vi "EAGLE GUI V3.vi"() -> ()   [LabVIEW 2015]
panel:
  in  "Tab Control":enum32{"Page 1", "Page 2", "Page 3"}(tab)
  in  "NewProcedure":bool caption="Boolean"
  in  "Ready":bool caption="Boolean"
  in  "EditRout":bool caption="Boolean"
  in  "Ready 2":bool caption="Boolean"
  in  "TabSelect":T1(radio)
  in  "Tab":enum32{"Page 1", "Page 2", "Page 3"}(tab)
  in  "EyeColor":u16(ring) caption="Eye Color:" items=["Brown", "Green", "Blue", "Black"]
  in  "SysLogPath":path caption="System Log Path:"
  in  "VideoPath":path caption="Video Output Path:"
  in  "PatientGender":enum32{"Male", "Female"}(radio) caption="Patient Gender:"
  in  "PatientAge":dbl caption="Patient Age:"
  in  "PatientName":string caption="Patient Name:"
  in  "Freeze":bool caption="Boolean"
  in  "Record":bool caption="Boolean"
  out "ProcStat":string caption="Procedure Data"
  out "SystemStatus":string caption="System Status"
  in  "OpenMenu":bool
  in  "Live Eye Image":T2(plugin-control)
  in  "Procedure Instructions":T3(ring)
  # "Aim the pupil to the center of the image\nMake sure the focus laser is in the \nbar Center"
  # "When Ready Press the GO Button"
  # "Procedure Parameters"
  # "System Configuration"
  # "Patient Statistics"
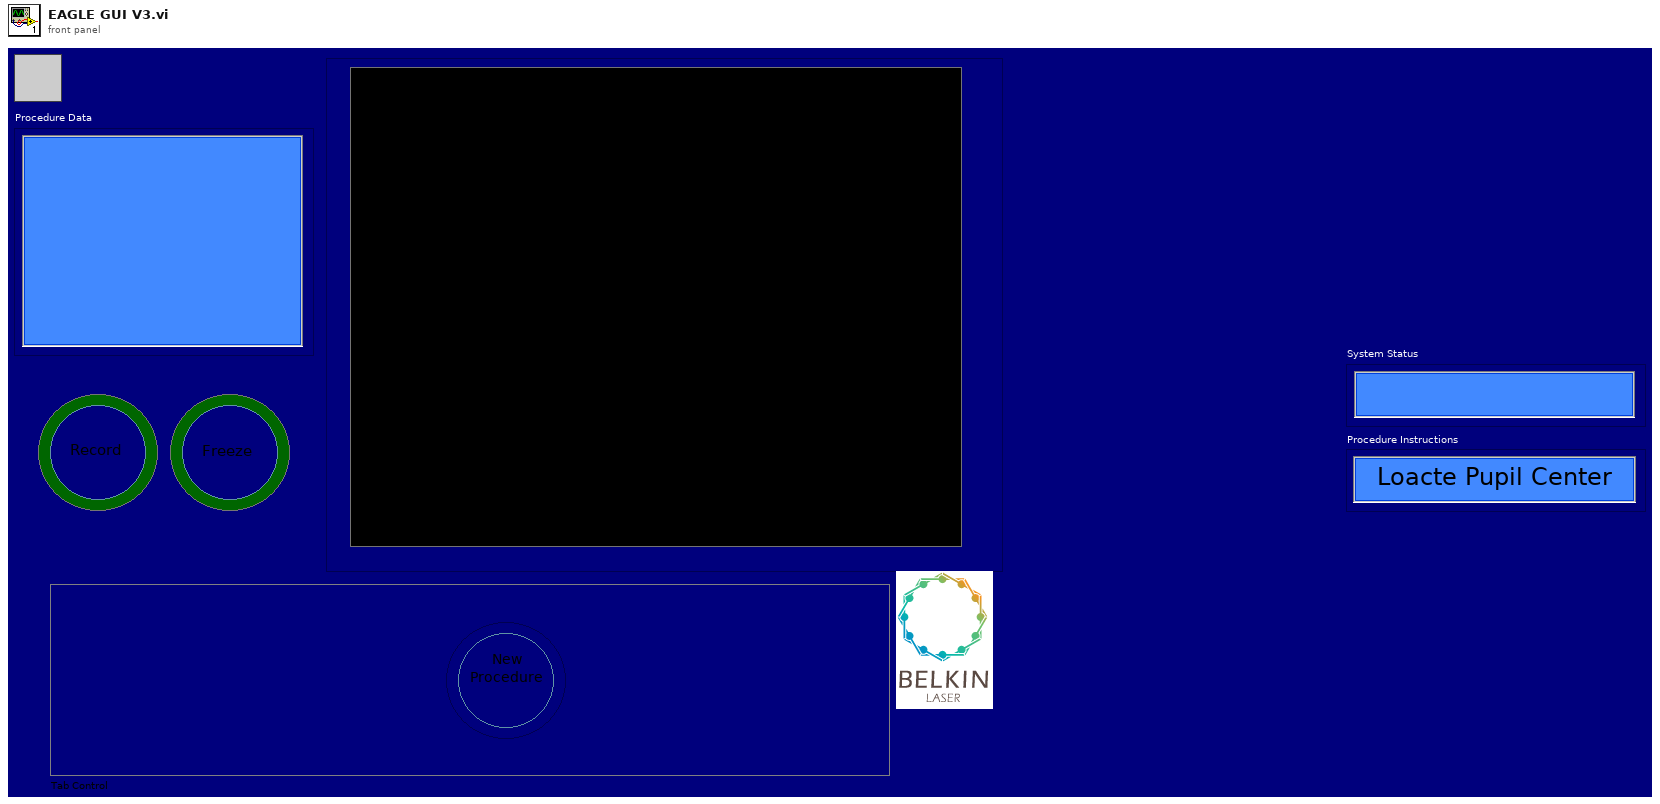
[diagram p1: front panel]
types:
  T1 = enum32{"Radio Selection 1", "Radio Selection 2", "Radio Selection 3"}
  T2 = typedef "IMAQ Image.ctl" = refnum<image>
  T3 = enum16{"Loacte Pupil Center", "Refine Distance", "CLick GO", "Process Finished"}
  T4 = typedef "LVRectTypeDef.ctl" = cluster{"Left":i16, "Top":i16, "Right":i16, "Bottom":i16}
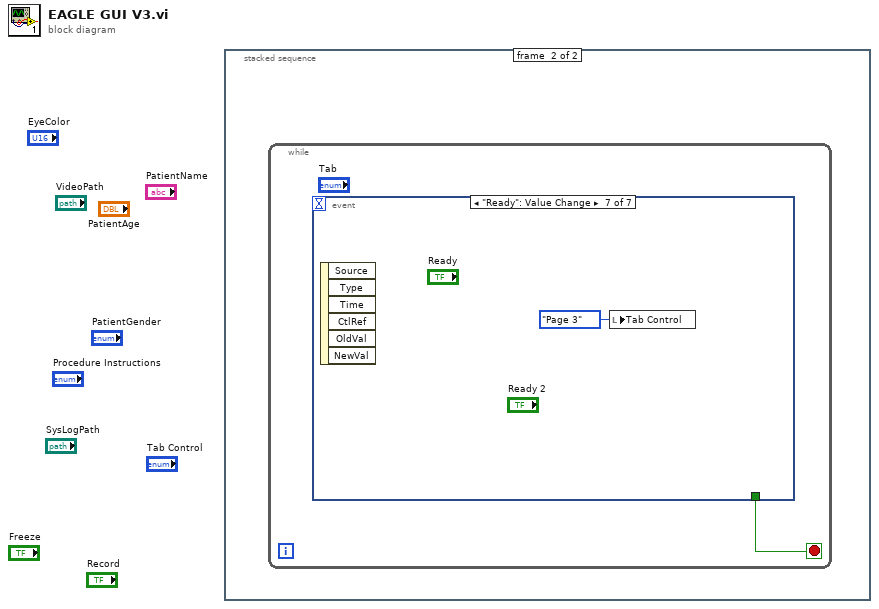
[diagram p0: block diagram]
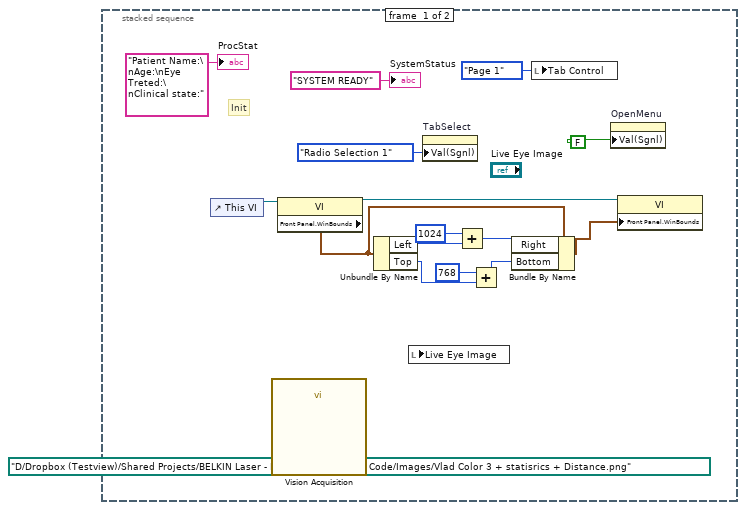
[diagram p2: hidden frame]
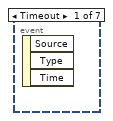
[diagram p3: hidden frame]
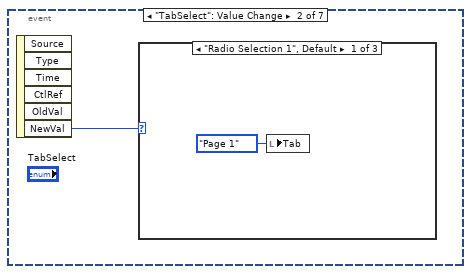
[diagram p4: hidden frame]
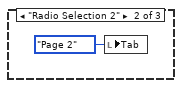
[diagram p5: hidden frame]
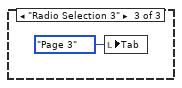
[diagram p6: hidden frame]
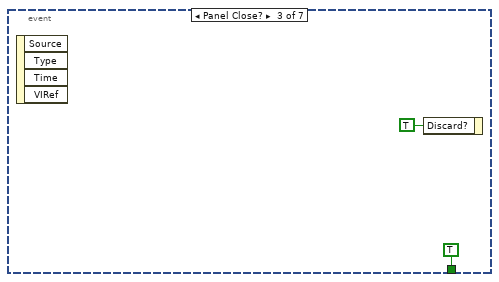
[diagram p7: hidden frame]
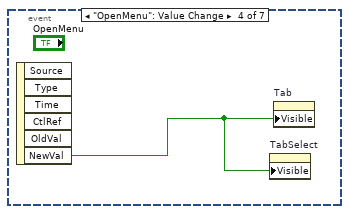
[diagram p8: hidden frame]
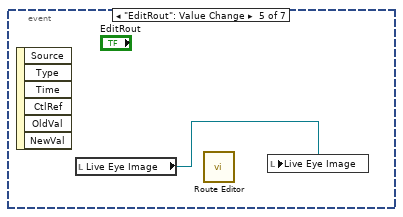
[diagram p9: hidden frame]
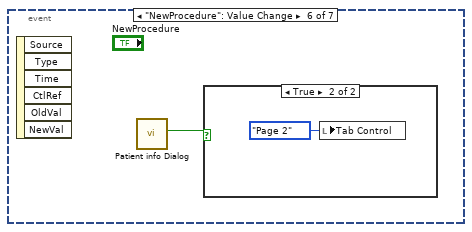
[diagram p10: hidden frame]
diagram:
  n1 = stacked-sequence {
    frame #0 {
      # "Init"
      n2 = control-ref of="This VI"() -> (w14:refnum<vi>)
      n3 = call "Vision Acquisition"("Image Path"=path "D:/Dropbox (Testview)/Shared Projects/BELKIN Laser - R&D/Software/DEMO Code/Images/Vlad Color 3 + statisrics + Distance.png") -> ()  [unwired: 25 in, 2 out]
      n4 = property class="VI"(reference=w14) -> (reference out=w13:refnum<vi>, "Front Panel.WinBounds"=w12:T4)  [unwired: 1 in, 1 out]
      n5 = Unbundle By Name(w12) -> ("Left"=w11:i16, "Top"=w6:i16)
      n6 = local read "Live Eye Image"() -> ()  [unwired: 1 in]
      n7 = property on="TabSelect" class="RadioBtnsControl (strict)"("Val(Sgnl)"=T1."Radio Selection 1" ("Value (Signaling)")) -> ()  [unwired: 2 in, 2 out]
      n8 = Add(x=i16 1024, y=w11) -> (x+y=w9:i16)
      n9 = Add(x=i16 768, y=w6) -> (x+y=w7:i16)
      n10 = Bundle By Name(cluster=w12, "Right"=w9, "Bottom"=w7) -> (w5:T4)
      n11 = local write "Tab Control"(enum32{"Page 1", "Page 2"}."Page 1" ("Tab Control")) -> ()
      n12 = property on="OpenMenu" class="Bool (strict)"("Val(Sgnl)"=FALSE ("Value (Signaling)")) -> ()  [unwired: 2 in, 2 out]
      n13 = property class="VI"(reference=w13, "Front Panel.WinBounds"=w5) -> ()  [unwired: 1 in, 2 out]
      "SystemStatus" <- "SYSTEM READY" ("SystemStatus")
      "ProcStat" <- "Patient Name:\nAge:\nEye Treted:\nClinical state:" ("ProcStat")
    }
    frame #1 {
      n14 = while {
        stop <- w17 stop-if-true
        n15 = event shown="[6] \"Ready\": Value Change" {
          selector: _ -> [_ _ _ _ _ _ _]
          dyn-events: _ -> [_ _ _ _ _ _ _]
          timeout: _ -> [_ _ _ _ _ _ _]
          tunnel: [_ _ TRUE _ _ _ _] -> w17
          event Timeout {
            n16 = event-data() -> ()  [unwired: 1 in, 3 out]
          }
          event "TabSelect": Value Change {
            n17 = event-data() -> ("NewVal"=w18:T1)  [unwired: 1 in, 5 out]
            n18 = case shown="\"Radio Selection 1\", Default" w18 {
              frame "Radio Selection 1", Default {
                n19 = local write "Tab"(enum32{"Page 1", "Page 2", "Page 3"}."Page 1" ("Tab")) -> ()
              }
              frame "Radio Selection 2" {
                n20 = local write "Tab"(enum32{"Page 1", "Page 2", "Page 3"}."Page 2" ("Tab")) -> ()
              }
              frame "Radio Selection 3" {
                n21 = local write "Tab"(enum32{"Page 1", "Page 2", "Page 3"}."Page 3" ("Tab")) -> ()
              }
            }
          }
          event Panel Close? {
            n22 = event-data() -> ()  [unwired: 1 in, 4 out]
            n23 = event-data("Discard?"=TRUE) -> ()  [unwired: 1 in, 1 out]
          }
          event "OpenMenu": Value Change {
            n24 = event-data() -> ("NewVal"=w24:bool)  [unwired: 1 in, 5 out]
            n25 = property on="TabSelect" class="RadioBtnsControl (strict)"("Visible"=w24) -> ()  [unwired: 2 in, 2 out]
            n26 = property on="Tab" class="TabCtl (strict)"("Visible"=w24) -> ()  [unwired: 2 in, 2 out]
          }
          event "EditRout": Value Change {
            n27 = event-data() -> ()  [unwired: 1 in, 6 out]
            n28 = local read "Live Eye Image"() -> (w25:T2)
            n29 = call "Route Editor.vi"() -> ()  [unwired: 11 in, 1 out]
            n30 = local write "Live Eye Image"(w25) -> ()
          }
          event "NewProcedure": Value Change {
            n31 = event-data() -> ()  [unwired: 1 in, 6 out]
            n32 = call "Patient info Dialog.vi"() -> ("OK"=w26:bool)  [unwired: 11 in]
            n33 = case shown="True" w26 {
              frame False {
              }
              frame True {
                n34 = local write "Tab Control"(enum32{"Page 1", "Page 2"}."Page 2" ("Tab Control")) -> ()
              }
            }
          }
          event "Ready": Value Change {
            n35 = event-data() -> ()  [unwired: 1 in, 6 out]
            n36 = local write "Tab Control"(enum32{"Page 1", "Page 2", "Page 3"}."Page 3" ("Tab Control")) -> ()
          }
        }
      }
    }
  }
